vi "AVS_GetNrOfDevices.vi"() -> (8 "Output Value":i32)   [LabVIEW 2016]
uses:
  libavs.so
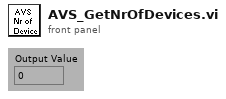
[diagram p1: front panel]
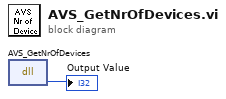
[diagram p0: block diagram]
diagram:
  n1 = dll-call lib="home/harini/tcs/ts_sedspectrometer/ss_sedspectrometer/VIs/libavs.so" fn="AVS_GetNrOfDevices"() -> ("return type"=→"Output Value":i32)  [unwired: 3 in, 2 out]
